vi "Pressure Sensor Test State.vi"(0 "GEA2 Reference Out":refnum<k24>, 5 "Queue in":refnum<queue>, 9 "Test Results in":T1, 11 "error in (no error)":errorcluster) -> (4 ".NET Refnum out":refnum<k24>, 10 "Test Results out":T1, 15 "error out":errorcluster)   [LabVIEW 2016]
doc: "This VI performs the LED test state."
uses:
  controls/Test Results.ctl
  C:/Program Files (x86)/National Instruments/LabVIEW 2016/examples/Design Patterns/Queued Message Handler/support/QMH Fundamentals - Message Cluster.ctl
  C:/Automation/DLLs/PC Dot Net/GeaCommunication.dll
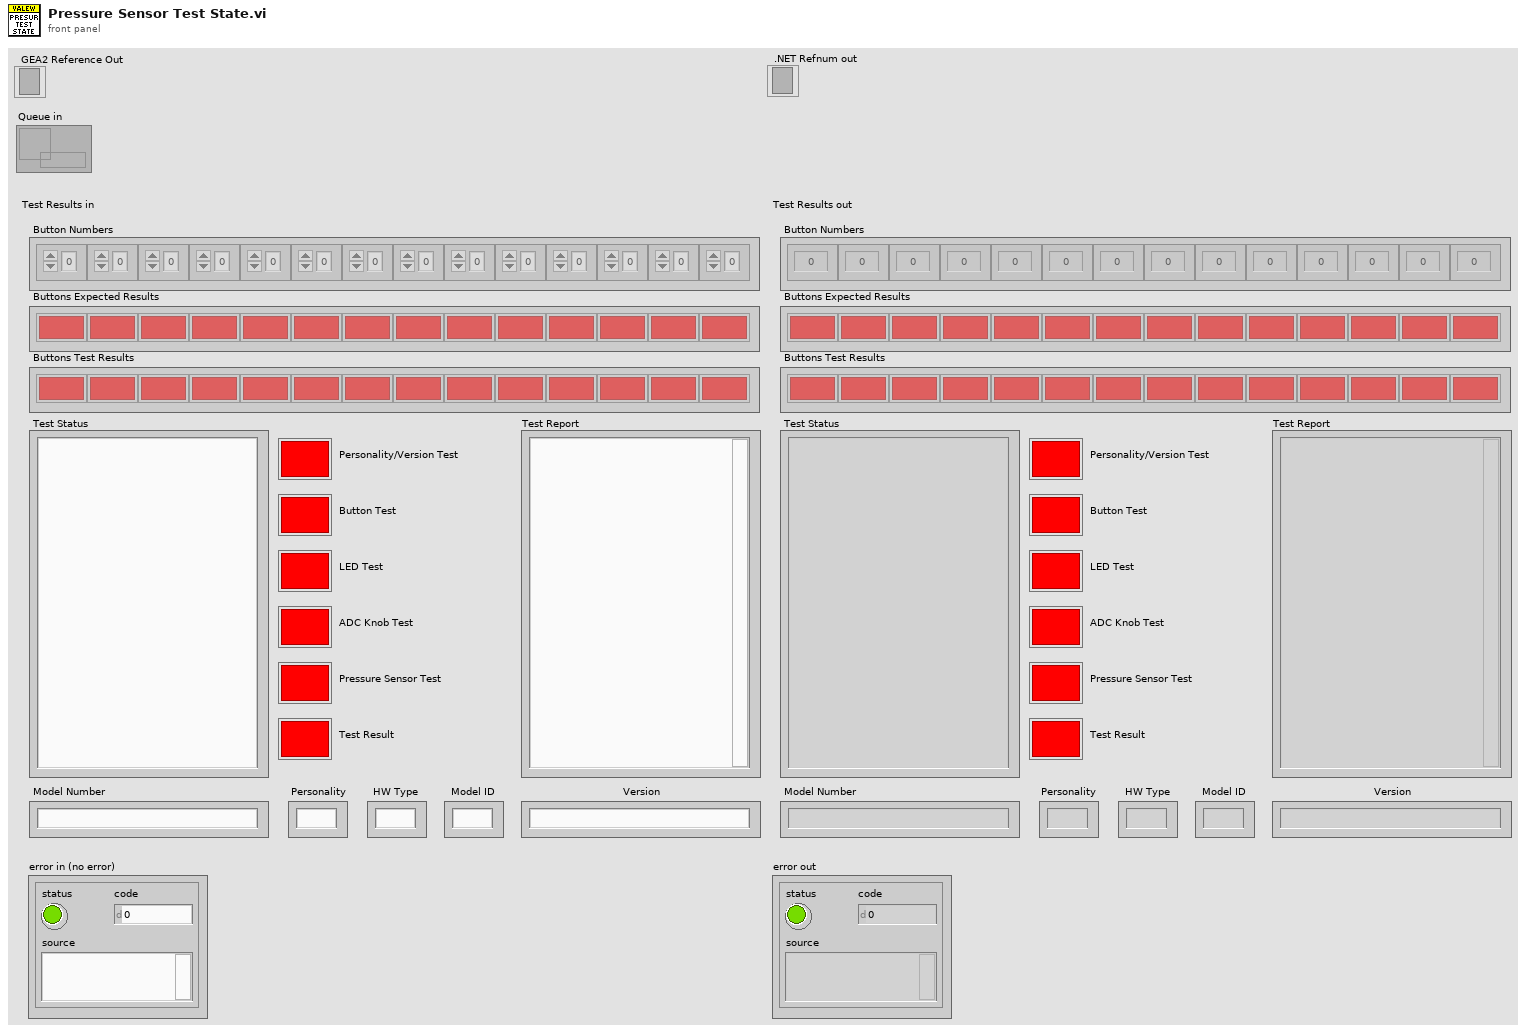
[diagram p1: front panel]
types:
  T1 = typedef "Test Results.ctl" = cluster{"Test Status":string, "Personality/Version Test ":bool, "Test Report":string, "Model Number":string, "Button Numbers":i32[], "Buttons Test Results":bool[], "Buttons Expected Results":bool[], "Model ID":string, "Personality":string, "HW Type":string, "Version":string, "Button Test":bool, "LED Test":bool, "ADC Knob Test":bool, "Pressure Sensor Test":bool, "Test Result":bool}
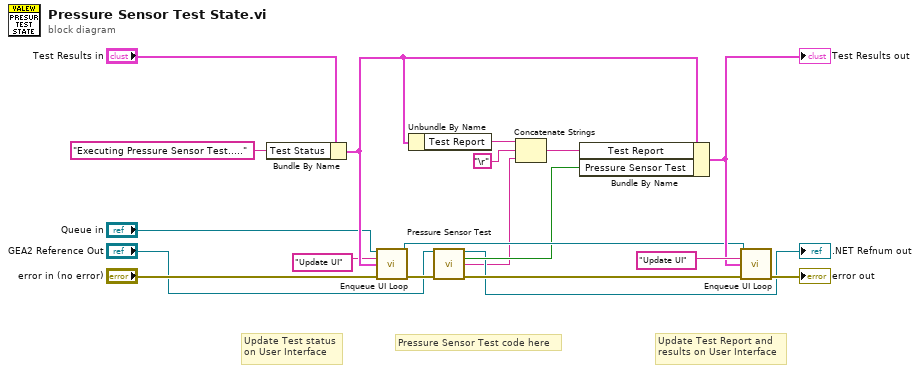
[diagram p0: block diagram]
diagram:
  # "Update Test Report and \nresults on User Interface"
  # "Pressure Sensor Test code here"
  # "Update Test status\non User Interface"
  n1 = Bundle By Name(cluster="Test Results in", "Test Status"="Executing Pressure Sensor Test.....") -> (w14:T1)
  n2 = call "Enqueue UI Loop.vi"("UI Que In"="Queue in", "Message"="Update UI", "Test Results"=w14, "error in (no error)"="error in (no error)") -> ("UI Queue Out"=w17:refnum<queue>, "error out"=w11:errorcluster)  [unwired: 10 in]
  n3 = Unbundle By Name(w14) -> ("Test Report"=w1:string)
  n4 = call "Pressure Sensor Test.vi"("GEA2 Reference In"="GEA2 Reference Out", "Error In"=w11) -> ("GEA2 Reference Out"=→".NET Refnum out":refnum<k24>, "Pass/Fail?"=w9:bool, "Report Text"=w4:string, "Error Out"=w15:errorcluster)  [unwired: 10 in]
  n5 = Concatenate Strings(w1, "\r", w4) -> (w3:string)
  n6 = Bundle By Name(cluster=w14, "Test Report"=w3, "Pressure Sensor Test"=w9) -> (w18:T1)
  "Test Results out" <- w18
  n7 = call "Enqueue UI Loop.vi"("UI Que In"=w17, "Message"="Update UI", "Test Results"=w18, "error in (no error)"=w15) -> ("error out"=→"error out":errorcluster)  [unwired: 10 in, 1 out]
